vi "插入数据.vi"(5 "data":variant, 7 "columns":string[](array[string]), 8 "error in (no error)":errorcluster, 10 "database":string, 11 "table":string) -> (0 "error out":errorcluster)   [LabVIEW 2016, in "斯坦道原位多参数.lvlib"]
uses:
  <vilib>/Utility/sysdir.llb/System Directory Type.ctl
  <vilib>/addons/database/Connection.llb/DB Tools Open Connec (String).vi
  <vilib>/addons/database/NI_Database_API.lvlib
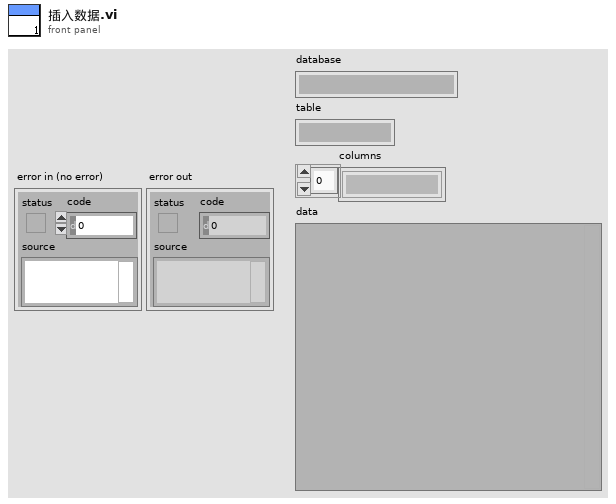
[diagram p1: front panel]
types:
  T1 = typedef "System Directory Type.ctl" = i32
  T2 = typedef "NI_Database_API.lvlib/Conn ObjectReference.ctl" = refnum<k1>
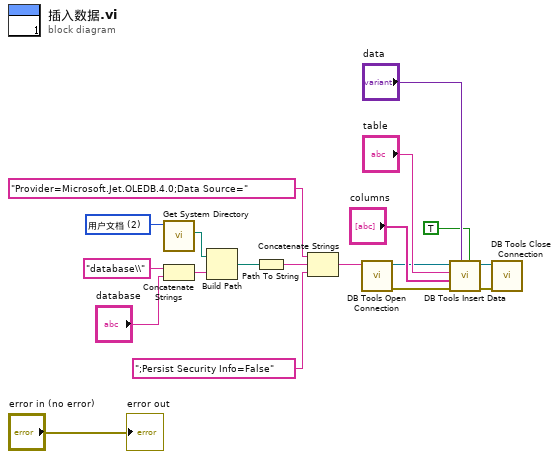
[diagram p0: block diagram]
diagram:
  w14 = T1 2 items=["用户目录"=0, "用户桌面"=1, "用户文档"=2, "用户应用程序数据"=3, "用户设置"=4, "用户临时目录"=5, "公共文档"=6, "公共应用程序数据"=7, "公共设置"=8, "公共缓存"=13, "系统核心库"=9, "系统安装库"=10, "应用程序文件"=11, "启动盘根目录"=12] ("system directory type")
  n1 = call <vilib>:"Get System Directory.vi"("system directory type"=w14) -> ("system directory"=w12:path)  [unwired: 10 in]
  n2 = Concatenate Strings("database\\" ("condition"), "database") -> (w6:string)
  n3 = Build Path(base path=w12, name or relative path=w6) -> (appended path=w11:path)
  n4 = Path To String(path=w11) -> (string=w10:string)
  n5 = Concatenate Strings("Provider=Microsoft.Jet.OLEDB.4.0;Data Source=" ("condition"), w10, ";Persist Security Info=False" ("condition")) -> (w8:string)
  n6 = call-poly <vilib>:"DB Tools Open Connection.vi"("connection information"=w8) -> ("error out"=w2:errorcluster, "connection reference"=w3:T2)  [unwired: 7 in]
  n7 = call <vilib>:"DB Tools Insert Data.vi"("create table? (F)"=TRUE, "data"="data", "error in (no error)"=w2, "columns"="columns", "table"="table", "connection reference"=w3) -> ("error out"=w18:errorcluster, "connection reference out"=w19:T2)  [unwired: 4 in]
  n8 = call <vilib>:"DB Tools Close Connection.vi"("error in (no error)"=w18, "connection reference"=w19) -> ()  [unwired: 5 in, 1 out]
  "error out" <- "error in (no error)"
